vi "Init GUI Objects.vi"(8 "Error In":errorcluster, 11 "GUI Object References":T1) -> (0 "Error Out":errorcluster)   [LabVIEW 2023, in "Error Manager.lvlib"]
doc: "This VI configures the \"look and feel\" of GUI objects, and sets their initial value (their contents)."
uses:
  Error Manager.lvlib
  GUI Object References (cluster).ctl
  Display Order Combo Box/Display Order Combo Box.lvclass
  Mark Selected Errors As Read Button/Mark Selected Errors As Read Button.lvclass
  Mark All Errors As Read Button/Mark All Errors As Read Button.lvclass
panel:
  out "Initial MCL Value":i32[](array[numeric])
  # "Development\nControls or indicators that are useful for development or testing, but which are not outputs of the VI."
  # "Input\nInputs to the VI"
  # "Output\nOutputs of the VI"
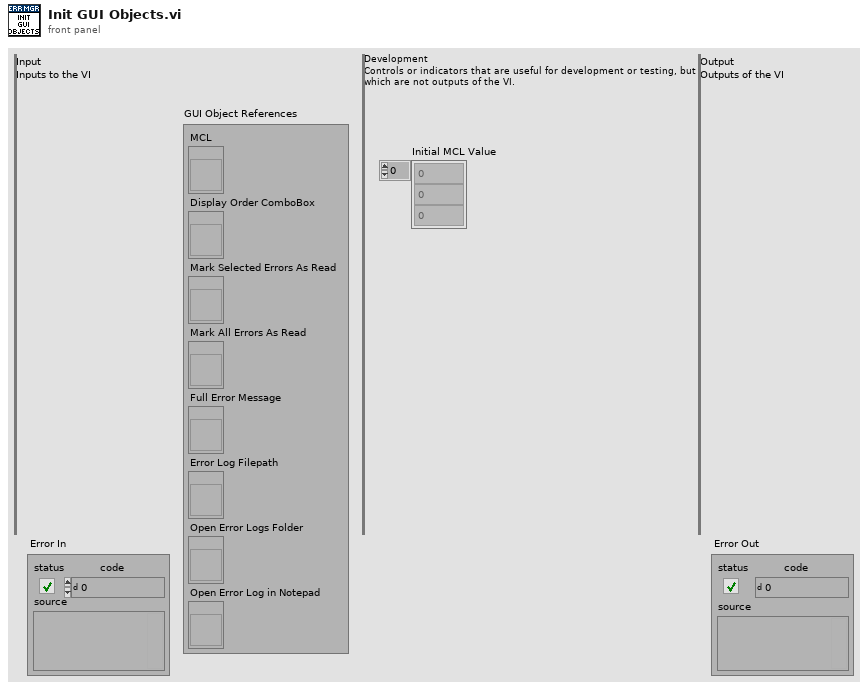
[diagram p1: front panel]
types:
  T1 = typedef "Error Manager.lvlib/GUI Object References (cluster).ctl" = cluster{"MCL":refnum<vi>, "Display Order ComboBox":refnum<vi>, "Mark Selected Errors As Read":refnum<vi>, "Mark All Errors As Read":refnum<vi>, "Full Error Message":refnum<vi>, "Error Log Filepath":refnum<vi>, "Open Error Logs Folder":refnum<vi>, "Open Error Log in Notepad":refnum<vi>}
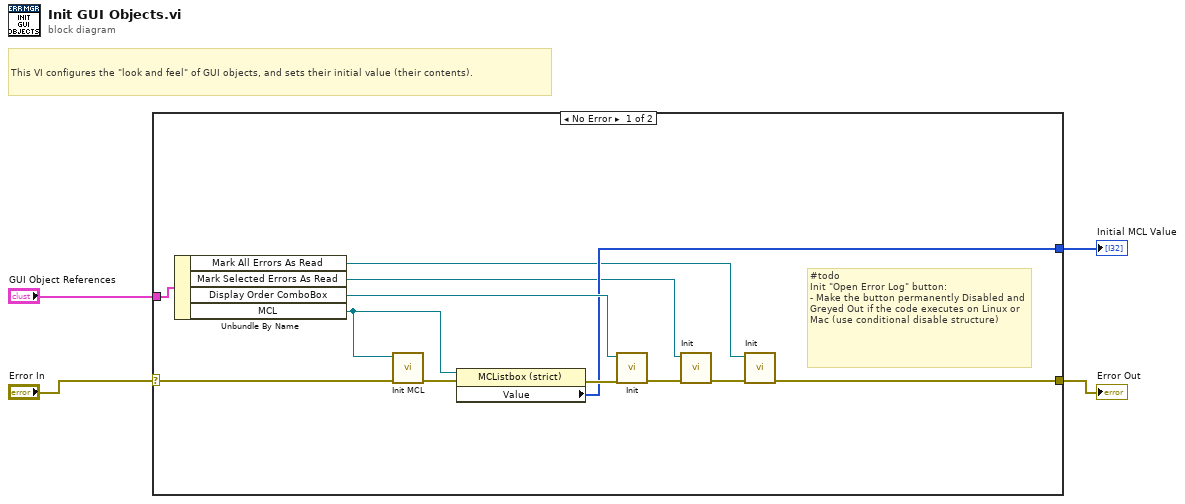
[diagram p0: block diagram]
diagram:
  # "This VI configures the \"look and feel\" of GUI objects, and sets their initial value (their contents)."
  n1 = case shown="No Error" "Error In" {
    selector: "Error In" -> [w16 w17]
    tunnel: [w6 w17] -> w3
    tunnel: "GUI Object References" -> [w15 _]
    tunnel: [w9 _] -> w1
    frame No Error {
      # "#todo\nInit \"Open Error Log\" button:\n- Make the button permanently Disabled and Greyed Out if the code executes on Linux or Mac (use conditional disable structure)"
      n2 = Unbundle By Name(w15) -> ("Mark All Errors As Read"=w5:refnum<vi>, "Mark Selected Errors As Read"=w7:refnum<vi>, "Display Order ComboBox"=w14:refnum<vi>, "MCL"=w12:refnum<vi>)
      n3 = call "Init MCL.vi"("error in (no error)"=w16, "MCL Reference"=w12) -> ("error out"=w13:errorcluster)  [unwired: 9 in]
      n4 = property class="MCListbox (strict)"(reference=w12, error in=w13) -> (error out=w10:errorcluster, "Value"=w9:i32[])  [unwired: 1 out]
      n5 = call "Init.vi"("error in (no error)"=w10, "ComboBox Ref"=w14) -> ("error out"=w8:errorcluster)  [unwired: 9 in]
      n6 = call "Init.vi"("error in (no error)"=w8, "Mark Selected Errors As Read Button Reference"=w7) -> ("error out"=w11:errorcluster)  [unwired: 9 in]
      n7 = call "Init.vi"("error in (no error)"=w11, "Mark All Errors As Read Button Reference"=w5) -> ("error out"=w6:errorcluster)  [unwired: 9 in]
    }
    frame Error {
    }
  }
  "Error Out" <- w3
  "Initial MCL Value" <- w1
